vi "Add Channel Data.vi"(4 "Inverted?":bool, 6 "Mean":bool, 8 "error in (no error)":errorcluster, 9 "Layer":enum16{"Top", "Bottom"}(ring), 10 "Channel Data":dbl[][](array[numeric])=array22x328[7216 elements], 11 "Graph Manager in":refnum<class "Graph Manager.lvclass">) -> (0 "error out":errorcluster, 2 "Channel ID":i32, 3 "Graph Manager out":refnum<class "Graph Manager.lvclass">)   [LabVIEW 2016, in "Graph Manager.lvclass"]
uses:
  Graph Manager.lvclass
  Graph Manager.lvclass/Graph Manager.ctl
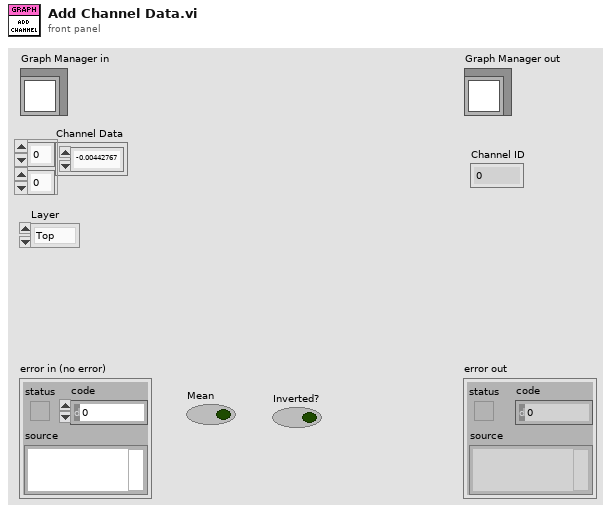
[diagram p1: front panel]
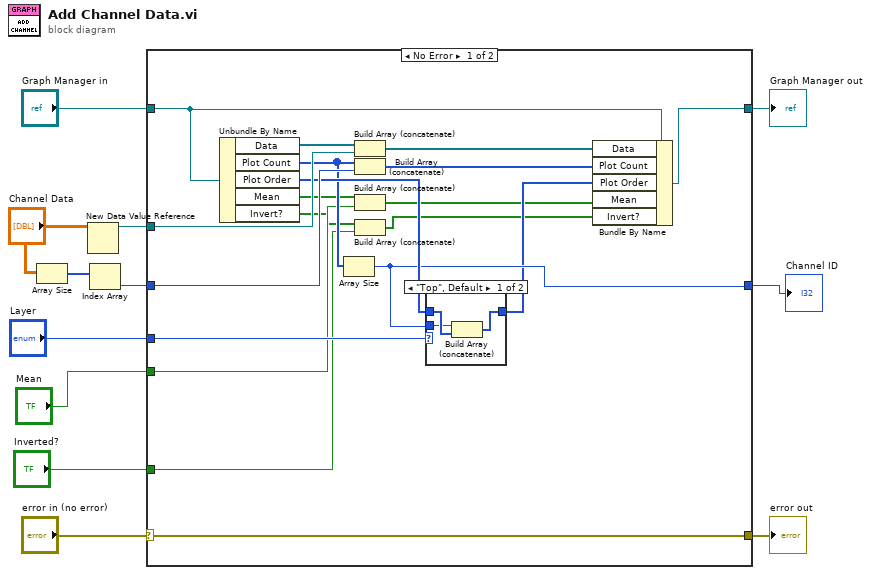
[diagram p0: block diagram]
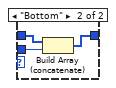
[diagram p2: hidden frame]
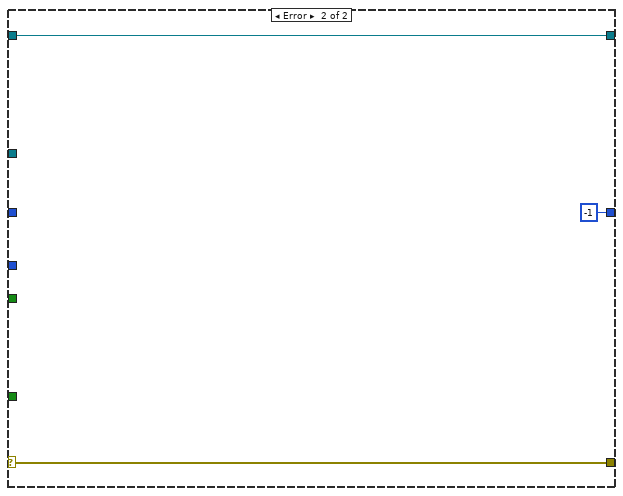
[diagram p3: hidden frame]
diagram:
  n1 = Array Size(array="Channel Data") -> (size(s)=w6:i32[])
  n2 = New Data Value Reference(data value="Channel Data") -> (data value reference=w8:refnum<data-value>)  [unwired: 1 in, 1 out]
  n3 = Index Array(array=w6) -> (element=w5:i32)  [unwired: 1 in]
  n4 = case shown="No Error" "error in (no error)" {
    selector: "error in (no error)" -> [w31 w40]
    tunnel: [w31 w40] -> w11
    tunnel: [w30 w39] -> w9
    tunnel: "Graph Manager in" -> [w29 w39]
    tunnel: w8 -> [w25 _]
    tunnel: w5 -> [w24 _]
    tunnel: [w20 -1] -> w4
    tunnel: "Layer" -> [w23 _]
    tunnel: "Mean" -> [w16 _]
    tunnel: "Inverted?" -> [w14 _]
    frame No Error {
      n5 = Unbundle By Name(w29) -> ("Data"=w28:refnum<data-value>[], "Plot Count"=w21:i32[], "Plot Order"=w22:i32[], "Mean"=w18:bool[], "Invert?"=w15:bool[])
      n6 = Array Size(array=w21) -> (size(s)=w20:i32)
      n7 = Build Array (concatenate)(w28, w25) -> (w27:refnum<data-value>[])
      n8 = Build Array (concatenate)(w21, w24) -> (w26:i32[])
      n9 = Build Array (concatenate)(w18, w16) -> (w17:bool[])
      n10 = Build Array (concatenate)(w15, w14) -> (w13:bool[])
      n11 = case shown="\"Top\", Default" w23 {
        tunnel: w22 -> [w34 w37]
        tunnel: w20 -> [w33 w36]
        tunnel: [w32 w35] -> w19
        frame "Top", Default {
          n12 = Build Array (concatenate)(w33, w34) -> (w32:i32[])
        }
        frame "Bottom" {
          n13 = Build Array (concatenate)(w37, w36) -> (w35:i32[])
        }
      }
      n14 = Bundle By Name(cluster=w29, "Data"=w27, "Plot Count"=w26, "Plot Order"=w19, "Mean"=w17, "Invert?"=w13) -> (w30:refnum<class "Graph Manager.lvclass">)
    }
    frame Error {
    }
  }
  "error out" <- w11
  "Graph Manager out" <- w9
  "Channel ID" <- w4
